vi "Power Output Abort Q Ops on Errors.vi"(8 "error in (no error)":errorcluster, 11 "Queue":refnum<queue>) -> (0 "error out":errorcluster)   [LabVIEW 2011]
uses:
  TypeDefs/Power Output Queue Cluster.ctl
  TypeDefs/Power Output Test Parameters.ctl
  TypeDefs/Power Output Stimulus Parameters.ctl
  TypeDefs/Power Output Measurement Parameters.ctl
  BPIMCore EXT/HW IO/DUTport.ctl
  BPIMCore EXT/HW IO/MeasMode.ctl
  BPIMCore EXT/HW IO/PIM Sweep Step Size.ctl
  TypeDefs/Power Output Display Parameters.ctl
  TypeDefs/Power Output Limit Parameters.ctl
  TypeDefs/Power Output Calibration State.ctl
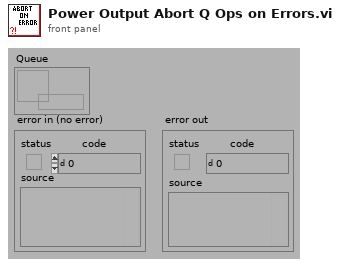
[diagram p1: front panel]
types:
  T1 = typedef "Power Output Test Parameters.ctl" = cluster{"Stimulus":T2, "Measurement":T3, "Display":T7, "Limit":T8, "Calibration":T9}
  T2 = typedef "Power Output Stimulus Parameters.ctl" = cluster{"Frequency Type":enum16{"Band Edges", "Custom"}, "Frequency Ranges":cluster{"Start (MHz)":dbl, "Stop (MHz)":dbl}[], "TX 1 Frequency (MHz)":cluster{"Min":dbl, "Max":dbl}, "TX 2 Frequency (MHz)":cluster{"Min":dbl, "Max":dbl}, "RX Frequency (MHz)":cluster{"Min":dbl, "Max":dbl}, "Pad Model Number":string, "Pad Serial Number":string, "Pad Values":dbl[][][]}
  T3 = typedef "Power Output Measurement Parameters.ctl" = cluster{"DUT Port":T4, "Direction":T5, "Frequency Step Size":T6}
  T4 = typedef "DUTport.ctl" = enum16{"Port 1", "Port 2"}
  T5 = typedef "MeasMode.ctl" = u16
  T6 = typedef "PIM Sweep Step Size.ctl" = u16
  T7 = typedef "Power Output Display Parameters.ctl" = cluster{"Frequency":cluster{"Min":dbl, "Max":dbl}, "Power":cluster{"Min":i32, "Max":i32}}
  T8 = typedef "Power Output Limit Parameters.ctl" = cluster{"Min Power (dBm)":dbl}
  T9 = typedef "Power Output Calibration State.ctl" = cluster{"Calibrated?":bool}
  T10 = cluster{string, "Power Verification Test Parameters":T1}
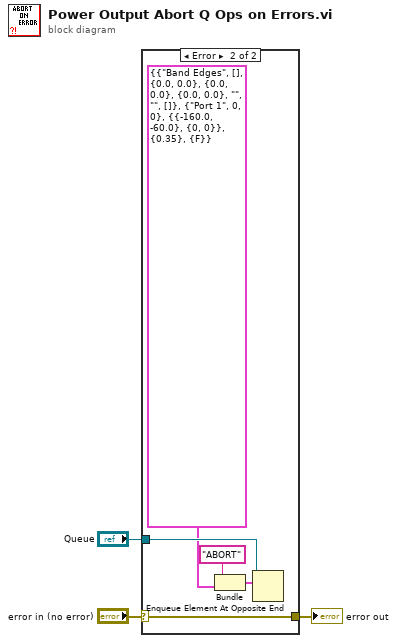
[diagram p0: block diagram]
diagram:
  n1 = case shown="Error" "error in (no error)" {
    selector: "error in (no error)" -> [w4 w9]
    tunnel: [w4 w9] -> w2
    tunnel: "Queue" -> [_ w7]
    frame No Error {
    }
    frame Error {
      n2 = Bundle("ABORT", "Power Verification Test Parameters"=T1 {"Stimulus"={"Frequency Type"=enum."Band Edges", "Frequency Ranges"=[], "TX 1 Frequency (MHz)"={"Min"=0.0, "Max"=0.0}, "TX 2 Frequency (MHz)"={"Min"=0.0, "Max"=0.0}, "RX Frequency (MHz)"={"Min"=0.0, "Max"=0.0}, "Pad Model Number"="", "Pad Serial Number"="", "Pad Values"=[]}, "Measurement"={"DUT Port"=enum."Port 1", "Direction"=0, "Frequency Step Size"=0}, "Display"={"Frequency"={"Min"=-160.0, "Max"=-60.0}, "Power"={"Min"=0, "Max"=0}}, "Limit"={"Min Power (dBm)"=0.35}, "Calibration"={"Calibrated?"=FALSE}}) -> (w5:T10)  [unwired: 1 out]
      n3 = Enqueue Element At Opposite End(queue=w7, element=w5) -> ()  [unwired: 1 in, 4 out]
    }
  }
  "error out" <- w2
